vi "Data Collect.vi"() -> ()   [LabVIEW 2015]
panel:
  out "布尔":bool
  out "子数组":string[](array[string])
  in  "Data Result":string[][](table)
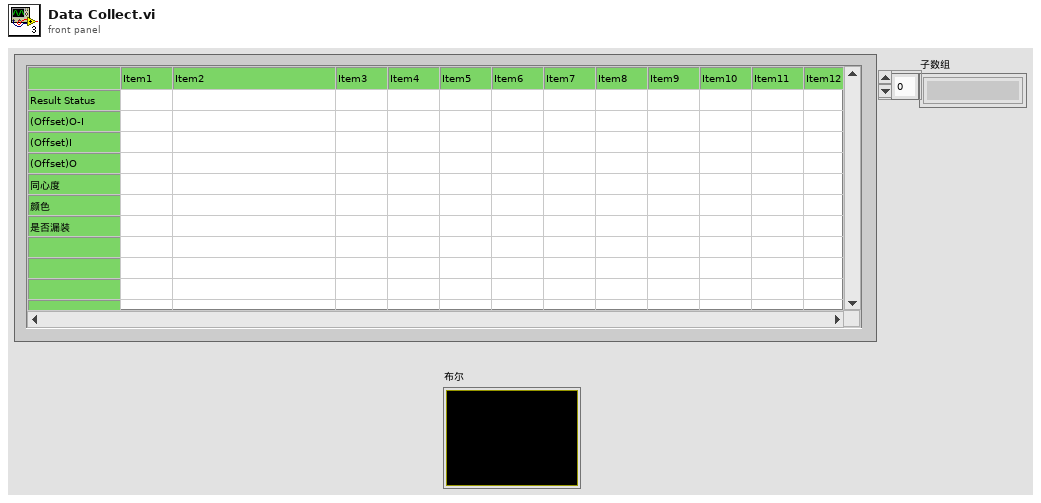
[diagram p1: front panel]
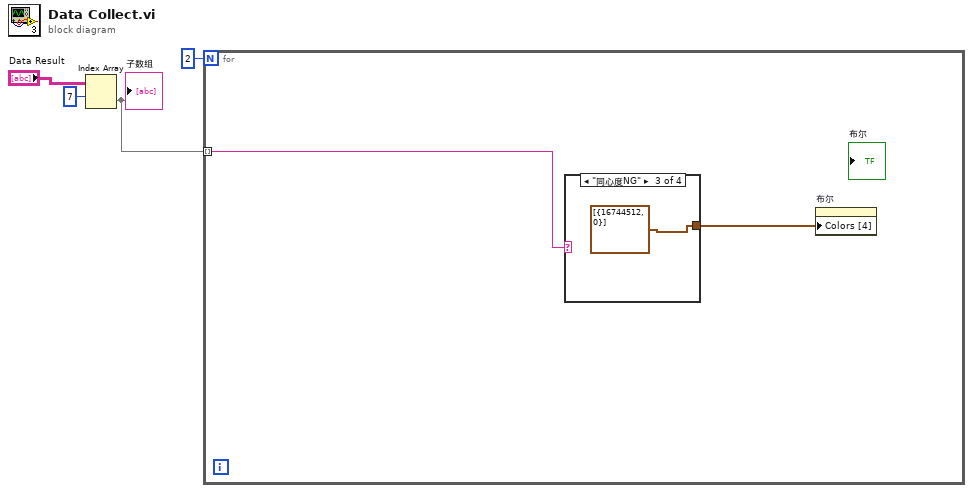
[diagram p0: block diagram]
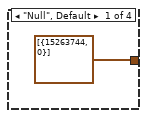
[diagram p2: hidden frame]
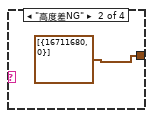
[diagram p3: hidden frame]
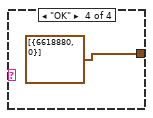
[diagram p4: hidden frame]
diagram:
  n1 = Index Array(array="Data Result", index (row)=7 ("索引 (行)")) -> (element=w2:string[])  [unwired: 1 in]
  "子数组" <- w2
  n2 = for {
    N: 2 -> [_]
    tunnel: w2 -> [w5] mode=indexing
    n3 = case shown="\"同心度NG\"" w5 {
      tunnel: [cluster{u32, u32}[] [{15263744, 0}] ("颜色[4]") cluster{u32, u32}[] [{16711680, 0}] ("颜色[4]") cluster{u32, u32}[] [{16744512, 0}] ("颜色[4]") cluster{u32, u32}[] [{6618880, 0}] ("颜色[4]")] -> w6
      frame "Null", Default {
      }
      frame "高度差NG" {
      }
      frame "同心度NG" {
      }
      frame "OK" {
      }
    }
    n4 = property on="布尔" class="Bool (严格)"("Colors [4]"=w6) -> ()  [unwired: 2 in, 2 out]
  }
